vi "AI Channel Page.vi"(8 "error in (no error)":errorcluster, 11 "Node Ptr":T1 format="%.0x") -> (0 "error out":errorcluster)   [LabVIEW 2013]
uses:
  <vilib>/K2Labs/HiLab API/Custom Device API/Controls/Custom Device Item Reference.ctl
  SubVIs/AI Terminal Configuration.ctl
  SubVIs/MeasurementType.ctl
  <vilib>/K2Labs/HiLab API/Custom Device API/Configuration/Item Properties/Get Item Property/Get Item Property.xnode
  <vilib>/K2Labs/HiLab API/Custom Device API/Configuration/Item Properties/Set Item Property/Set Item Property.xnode
  <vilib>/K2Labs/HiLab API/Custom Device API/Custom Device API Library.lvlib
  <vilib>/Utility/miscctls.llb/LVOutOfRangeActionTypeDef.ctl
panel:
  in  "NAME":string caption="名称"
  in  "UNITS":string caption="Units"
  in  "DESCRIPTION":string caption="描述"
  in  "ScaleOffset":dbl caption="缩放偏移量"
  in  "ScaleFactor":dbl caption="缩放因素"
  in  "MeasurementType":T2(ring) caption="测量类型"
  in  "Terminal Configuration":T3 caption="采集接线端配置"
  in  "Min":dbl=-10.0 caption="最小值" format="%#g"
  in  "Max":dbl=10.0 caption="最大值" format="%#g"
  in  "DEFAULTVALUE":dbl caption="默认值"
  in  "Physical Channel":string caption="物理通道"
  # "AI Channel"
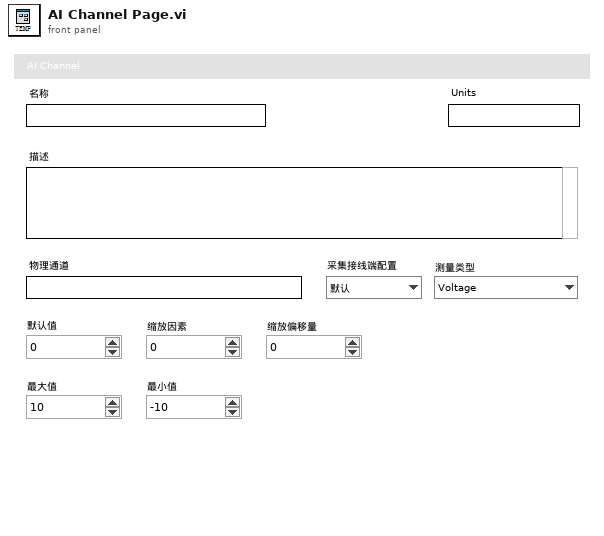
[diagram p1: front panel]
types:
  T1 = typedef "Custom Device API Library.lvlib/Custom Device Item Reference.ctl" = u64
  T2 = enum16{"Voltage", "Current", "More:Voltage:Custom with Excitation", "More:Current:Custom with Excitation", "Frequency", "Period", "Resistance", "Temperature:Thermocouple", "Temperature:Thermistor", "Temperature:RTD", "Temperature:Built-in Sensor", "Strain Gage"}
  T3 = typedef "AI Terminal Configuration.ctl" = enum16{"默认", "RSE", "NRSE", "差分", "伪差分"}
  T4 = typedef "MeasurementType.ctl" = enum16{"Voltage", "Current", "More:Voltage:Custom with Excitation", "More:Current:Custom with Excitation", "Frequency", "Period", "Resistance", "Temperature:Thermocouple", "Temperature:Thermistor", "Temperature:RTD", "Temperature:Built-in Sensor", "Strain Gage"}
  T5 = typedef "LVOutOfRangeActionTypeDef.ctl" = cluster{"Out of Range Action Minimum":u8, "Out of Range Action Maximum":u8, "Out of Range Action Increment":u8}
  T6 = typedef "Custom Device API Library.lvlib/Custom Device System Configuration Command Type.ctl" = enum16{"Default", "Menu Selected", "Shutdown", "Dynamic button pressed"}
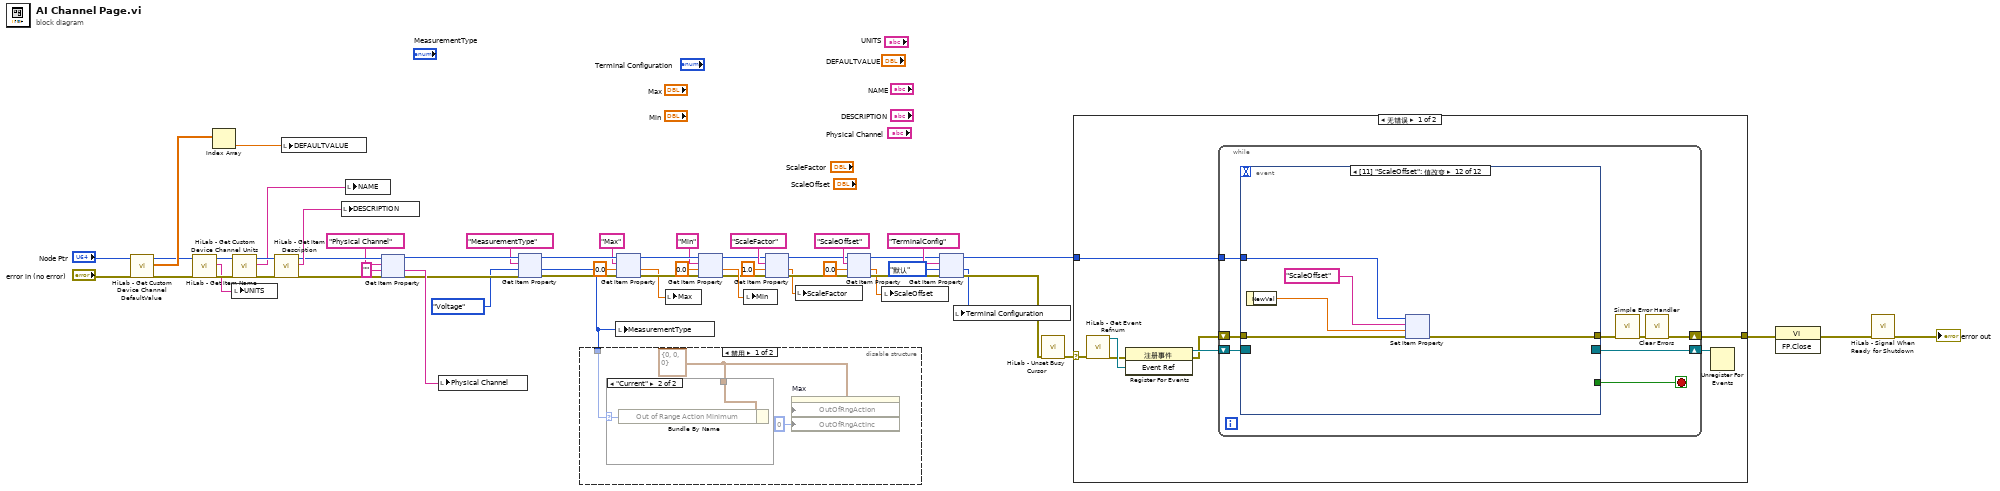
[diagram p0: block diagram]
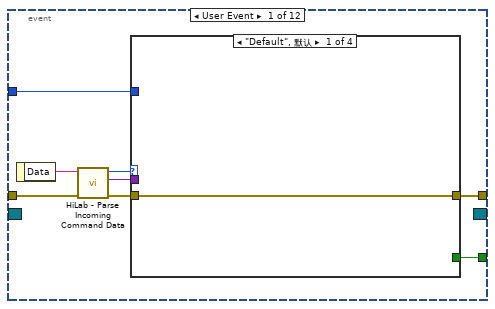
[diagram p4: hidden frame]
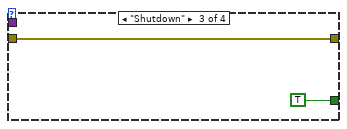
[diagram p6: hidden frame]
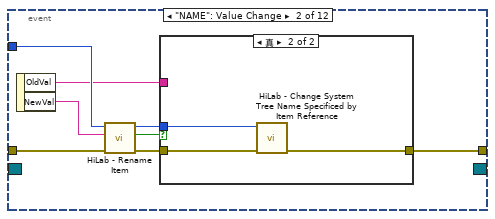
[diagram p8: hidden frame]
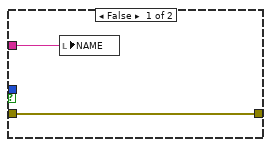
[diagram p9: hidden frame]
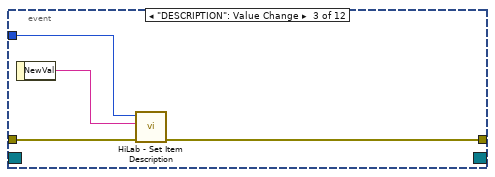
[diagram p10: hidden frame]
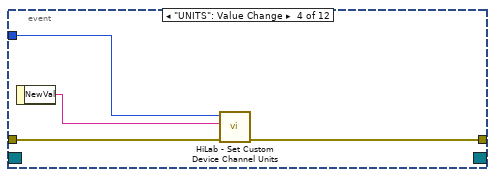
[diagram p11: hidden frame]
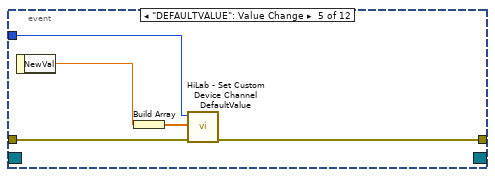
[diagram p12: hidden frame]
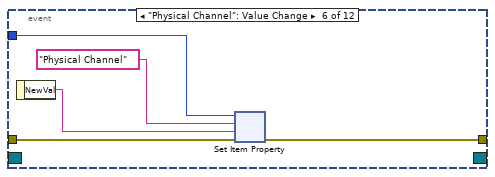
[diagram p13: hidden frame]
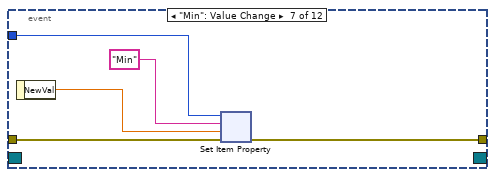
[diagram p14: hidden frame]
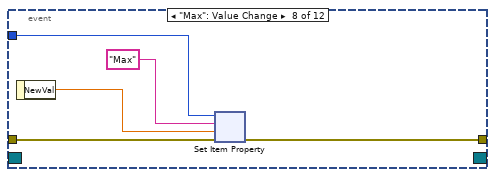
[diagram p15: hidden frame]
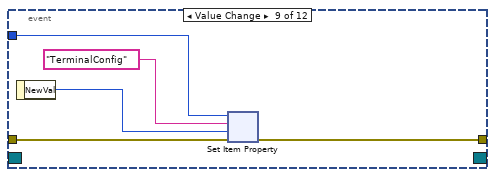
[diagram p16: hidden frame]
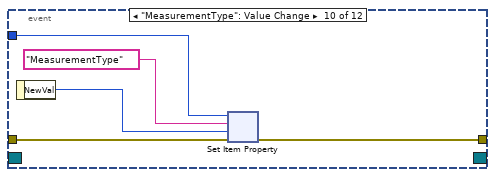
[diagram p17: hidden frame]
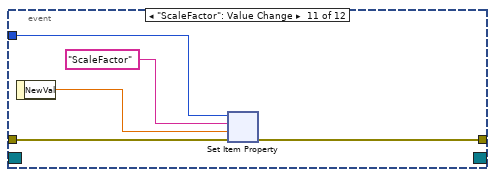
[diagram p18: hidden frame]
diagram:
  n1 = call <vilib>:"HiLab - Get Custom Device Channel DefaultValue.vi"("error in (no error)"="error in (no error)", "Channel Ref in"="Node Ptr") -> ("error out"=w16:errorcluster, "DefaultValue"=w41:dbl[], "Channel Ref out"=w17:T1)  [unwired: 6 in, 1 out]
  n2 = call <vilib>:"HiLab - Get Custom Device Channel Units.vi"("error in (no error)"=w16, "Channel Ref in"=w17) -> ("error out"=w14:errorcluster, "Units"=w13:string, "Channel Ref out"=w15:T1)  [unwired: 7 in]
  n3 = Index Array(array=w41) -> (element=w39:dbl)  [unwired: 1 in]
  n4 = local write "UNITS"(w13) -> ()
  n5 = call <vilib>:"HiLab - Get Item Name.vi"("error in (no error)"=w14, "Item Ref in"=w15) -> ("error out"=w53:errorcluster, "Name"=w51:string, "Item Ref out"=w54:T1)  [unwired: 6 in, 1 out]
  n6 = call <vilib>:"HiLab - Get Item Description.vi"("error in (no error)"=w53, "Item Ref in"=w54) -> ("error out"=w45:errorcluster, "Discription"=w52:string, "Item Ref out"=w46:T1)  [unwired: 6 in, 1 out]
  n7 = local write "DEFAULTVALUE"(w39) -> ()
  n8 = local write "DESCRIPTION"(w52) -> ()
  n9 = local write "NAME"(w51) -> ()
  n10 = xnode "Get Item Property"("Item Ref in"=w46, "Property Name"="Physical Channel", "Default Value"="", "error in (no error)"=w45) -> ("Item Ref out"=w38:T1, "Value"=w40:string, "error out"=w37:errorcluster)  [unwired: 1 out]
  n11 = local write "Physical Channel"(w40) -> ()
  n12 = xnode "Get Item Property"("Item Ref in"=w38, "Property Name"="MeasurementType", "Default Value"=MeasurementType."Voltage" ("MeasurementType"), "error in (no error)"=w37) -> ("Item Ref out"=w35:T1, "Value"=w28:T4, "error out"=w36:errorcluster)  [unwired: 1 out]
  n13 = disable-structure shown="禁用" {
    disable-tunnel: w28 -> [w57 _]
    frame Disabled {
      w55 = T5 {"Out of Range Action Minimum"=0, "Out of Range Action Maximum"=0, "Out of Range Action Increment"=0} ("对超出界限的值的响应")
      n14 = case shown="\"Current\"" w57 {
        selector: w57 -> [_ w59]
        tunnel: w55 -> [_ w58]
        frame "Voltage", Default {
        }
        frame "Current" {
          n15 = Bundle By Name(cluster=w58, "Out of Range Action Minimum"=w59) -> ()  [unwired: 1 out]
        }
      }
      n16 = property on="Max" class="DigNum (严格)"("OutOfRngAction"=w55, "OutOfRngActInc"=u8 0 ("对超出界限的值的响应:增量")) -> ()  [unwired: 2 in, 2 out]
    }
    frame Enabled {
    }
  }
  n17 = local write "MeasurementType"(w28) -> ()
  n18 = xnode "Get Item Property"("Item Ref in"=w35, "Property Name"="Max", "Default Value"=0.0, "error in (no error)"=w36) -> ("Item Ref out"=w34:T1, "Value"=w27:dbl, "error out"=w33:errorcluster)  [unwired: 1 out]
  n19 = local write "Max"(w27) -> ()
  n20 = xnode "Get Item Property"("Item Ref in"=w34, "Property Name"="Min", "Default Value"=0.0, "error in (no error)"=w33) -> ("Item Ref out"=w6:T1, "Value"=w26:dbl, "error out"=w7:errorcluster)  [unwired: 1 out]
  n21 = local write "Min"(w26) -> ()
  n22 = xnode "Get Item Property"("Item Ref in"=w6, "Property Name"="ScaleFactor", "Default Value"=1.0, "error in (no error)"=w7) -> ("Item Ref out"=w8:T1, "Value"=w2:dbl, "error out"=w5:errorcluster)  [unwired: 1 out]
  n23 = local write "ScaleFactor"(w2) -> ()
  n24 = xnode "Get Item Property"("Item Ref in"=w8, "Property Name"="ScaleOffset", "Default Value"=0.0, "error in (no error)"=w5) -> ("Item Ref out"=w4:T1, "Value"=w1:dbl, "error out"=w3:errorcluster)  [unwired: 1 out]
  n25 = local write "ScaleOffset"(w1) -> ()
  n26 = xnode "Get Item Property"("Item Ref in"=w4, "Property Name"="TerminalConfig", "Default Value"=AI_Terminal_Configuration."默认" ("Terminal Configuration"), "error in (no error)"=w3) -> ("Item Ref out"=w23:T1, "Value"=w24:T3, "error out"=w25:errorcluster)  [unwired: 1 out]
  n27 = local write "Terminal Configuration"(w24) -> ()
  n28 = call <vilib>:"HiLab - Unset Busy Cursor.vi"("error in (no error)"=w25) -> ("error out"=w50:errorcluster)  [unwired: 10 in]
  n29 = case shown="无错误" w50 {
    selector: w50 -> [w62 w346]
    tunnel: [w67 w346] -> w49
    tunnel: w23 -> [w66 _]
    frame No Error {
      n30 = call <vilib>:"HiLab - Get Event Refnum.vi"("error in (no error)"=w62) -> ("error out"=w60:errorcluster, "Event Ref"=w61:refnum<user-event>)  [unwired: 9 in]
      n31 = register-events(error in=w60, w61) -> (reference out=w65:refnum<event-registration>, error out=w63:errorcluster)  [unwired: 1 in]
      n32 = while {
        shift-right: [w71] -> w67
        shift-left: w63 -> [w74]
        tunnel: w66 -> [w70]
        shift-right: [w68] -> w64
        shift-left: w65 -> [w69]
        stop <- w75 stop-if-true
        n33 = event shown="[11] \"ScaleOffset\": 值改变" {
          selector: w69 -> [_ _ _ _ _ _ _ _ _ _ _ _]
          dyn-events: [_ _ _ _ _ _ _ _ _ _ _ _] -> w68
          timeout: _ -> [_ _ _ _ _ _ _ _ _ _ _ _]
          tunnel: [w77 _ _ _ _ _ _ _ _ _ _ _] -> w75
          tunnel: w74 -> [w82 w95 w104 w107 w113 w116 w149 w182 w217 w250 w283 w316]
          tunnel: [w78 w89 w102 w106 w112 w115 w148 w181 w216 w249 w282 w315] -> w73
          tunnel: w70 -> [w79 w96 w105 w108 w114 w119 w152 w185 w218 w251 w284 w317]
          event User Event {
            n34 = event-data() -> ("Data"=w83:string)  [unwired: 1 in]
            n35 = call <vilib>:"HiLab - Parse Incoming Command Data.vi"("error in (no error)"=w82, "Incoming Command Data"=w83) -> ("error out"=w80:errorcluster, "Data"=w76:variant, "Actions"=w81:T6)  [unwired: 7 in]
            n36 = case shown="\"Default\", 默认" w81 {
              tunnel: w80 -> [w84 w85 w87 w88]
              tunnel: w79 -> [_ _ _ _]
              tunnel: [w84 w85 w87 w88] -> w78
              tunnel: [_ _ TRUE _] -> w77
              tunnel: w76 -> [_ _ _ _]
              frame "Default", Default {
              }
              frame "Menu Selected" {
              }
              frame "Shutdown" {
              }
              frame "Dynamic button pressed" {
              }
            }
          }
          event "NAME": Value Change {
            n37 = event-data() -> ("OldVal"=w92:string, "NewVal"=w94:string)  [unwired: 1 in]
            n38 = call <vilib>:"HiLab - Rename Item.vi"("error in (no error)"=w95, "New Name"=w94, "Item Ref in"=w96) -> ("error out"=w90:errorcluster, "Success?"=w93:bool, "Item Ref out"=w91:T1)  [unwired: 6 in]
            n39 = case shown="真" w93 {
              tunnel: w92 -> [w98 _]
              tunnel: w91 -> [_ w101]
              tunnel: w90 -> [w97 w100]
              tunnel: [w97 w99] -> w89
              frame False {
                n40 = local write "NAME"(w98) -> ()
              }
              frame True {
                n41 = call <vilib>:"HiLab - Change System Tree Name Specificed by Item Reference.vi"("error in (no error)"=w100, "Item Ref in"=w101) -> ("error out"=w99:errorcluster)  [unwired: 8 in, 1 out]
              }
            }
          }
          event "DESCRIPTION": Value Change {
            n42 = event-data() -> ("NewVal"=w103:string)  [unwired: 1 in]
            n43 = call <vilib>:"HiLab - Set Item Description.vi"("error in (no error)"=w104, "Discription"=w103, "Item Ref in"=w105) -> ("error out"=w102:errorcluster)  [unwired: 6 in, 2 out]
          }
          event "UNITS": Value Change {
            n44 = event-data() -> ("NewVal"=w109:string)  [unwired: 1 in]
            n45 = call <vilib>:"HiLab - Set Custom Device Channel Units.vi"("error in (no error)"=w107, "Units"=w109, "Channel Ref in"=w108) -> ("error out"=w106:errorcluster)  [unwired: 7 in, 1 out]
          }
          event "DEFAULTVALUE": Value Change {
            n46 = event-data() -> ("NewVal"=w110:dbl)  [unwired: 1 in]
            n47 = Build Array(w110) -> (w111:dbl[])
            n48 = call <vilib>:"HiLab - Set Custom Device Channel DefaultValue.vi"("error in (no error)"=w113, "DefaultValue"=w111, "Channel Ref in"=w114) -> ("error out"=w112:errorcluster)  [unwired: 7 in, 1 out]
          }
          event "Physical Channel": Value Change {
            n49 = event-data() -> ("NewVal"=w117:string)  [unwired: 1 in]
            n50 = xnode "Set Item Property"("Item Ref in"=w119, "error in (no error)"=w116, "Property Name"="Physical Channel", "Value"=w117) -> ("error out"=w115:errorcluster)  [unwired: 2 out]
          }
          event "Min": Value Change {
            n51 = event-data() -> ("NewVal"=w150:dbl)  [unwired: 1 in]
            n52 = xnode "Set Item Property"("Item Ref in"=w152, "error in (no error)"=w149, "Property Name"="Min", "Value"=w150) -> ("error out"=w148:errorcluster)  [unwired: 2 out]
          }
          event "Max": Value Change {
            n53 = event-data() -> ("NewVal"=w183:dbl)  [unwired: 1 in]
            n54 = xnode "Set Item Property"("Item Ref in"=w185, "error in (no error)"=w182, "Property Name"="Max", "Value"=w183) -> ("error out"=w181:errorcluster)  [unwired: 2 out]
          }
          event Value Change {
            n55 = event-data() -> ("NewVal"=w215:T3)  [unwired: 1 in]
            n56 = xnode "Set Item Property"("Item Ref in"=w218, "error in (no error)"=w217, "Property Name"="TerminalConfig", "Value"=w215) -> ("error out"=w216:errorcluster)  [unwired: 2 out]
          }
          event "MeasurementType": Value Change {
            n57 = event-data() -> ("NewVal"=w248:T2)  [unwired: 1 in]
            n58 = xnode "Set Item Property"("Item Ref in"=w251, "error in (no error)"=w250, "Property Name"="MeasurementType", "Value"=w248) -> ("error out"=w249:errorcluster)  [unwired: 2 out]
          }
          event "ScaleFactor": Value Change {
            n59 = event-data() -> ("NewVal"=w281:dbl)  [unwired: 1 in]
            n60 = xnode "Set Item Property"("Item Ref in"=w284, "error in (no error)"=w283, "Property Name"="ScaleFactor", "Value"=w281) -> ("error out"=w282:errorcluster)  [unwired: 2 out]
          }
          event "ScaleOffset": Value Change {
            n61 = event-data() -> ("NewVal"=w314:dbl)  [unwired: 1 in]
            n62 = xnode "Set Item Property"("Item Ref in"=w317, "error in (no error)"=w316, "Property Name"="ScaleOffset", "Value"=w314) -> ("error out"=w315:errorcluster)  [unwired: 2 out]
          }
        }
        n63 = call <vilib>:"Simple Error Handler.vi"("error in (no error)"=w73) -> ("error out"=w72:errorcluster)  [unwired: 4 in, 4 out]
        n64 = call <vilib>:"Clear Errors.vi"("error in (no error)"=w72) -> ("error out"=w71:errorcluster)  [unwired: 6 in]
      }
      n65 = Unregister For Events(event registration refnum=w64) -> ()  [unwired: 1 in, 1 out]
    }
    frame Error {
    }
  }
  n66 = invoke class="VI" method="FP.Close"(error in=w49) -> (error out=w48:errorcluster)  [unwired: 2 in, 2 out]
  n67 = call <vilib>:"HiLab - Signal When Ready for Shutdown.vi"("error in (no error)"=w48) -> ("error out"=→"error out":errorcluster)  [unwired: 10 in]
